vi "Source A.vi"() -> ()   [LabVIEW 2016, in "beamline sections.lvlib"]
doc: "This vi allows the user to control the beamline elements on the high voltage deck. It uses the GRoup3 controllers to access all three high voltage decks. The preacc and injector image faraday cup are controlled by the low end compact rio"
uses:
  controls/beamline sections.lvlib
  controls/SCA steerers.ctl
  save load/saveloadprev.ctl
  cRIO code/SCA/controls/SCA broadcast status.ctl
  save load/SaveLoad.lvlib
panel:
  in  "Tab Control":T1(tab)
  in  "Preview-Save-Load":T2
  out "Boolean":bool
  in  "Oven i":dbl
  in  "Y Steerer":dbl(slide) scale=-500.0..500.0
  in  "Pre-Acc":dbl(slide) scale=0.0..63.0
  in  "Einzel 2":dbl(slide) scale=0.0..10.0
  in  "X Steerer":dbl(slide) scale=-500.0..500.0
  in  "Einzel 1":dbl(slide) scale=0.0..12.0
  in  "Extractor":dbl(slide) scale=0.0..26.0
  in  "Immersion Lens":dbl(slide) scale=0.0..1.0
  out "Einzel 2 display":bool
  out "Cathode display":bool
  out "Oven display":bool
  out "Einzel 1 display":bool
  out "Immersion lens display":bool
  out "Steerer display":bool
  out "Pre acc display":bool=TRUE
  in  "Cathode V":dbl(slide) scale=0.0..12.0
  out "Cathode  cluster":T3 {"Cathode" format="%#_3g"; "Cathode\nVoltage" format="%#.2g"; "Cathode \nCurrent" format="%#.2g"}
  out "Extractor  cluster":T4 {"Extractor" format="%#_3g"; "Extractor \nVoltage" format="%#.2g"; "Extractor\n Current" format="%#.2g"}
  out "Immersion Lens  cluster":T5 {"Immersion Lens" format="%#_3g"; "Immersion Lens\nCurrent" format="%#.2g"; "Immersion Lens\nVoltage" format="%#.2g"}
  in  "stop":bool
  out "Oven cluster":T6 {"Oven V" format="%#.2g"; "Oven power" format="%#.2g"; "Oven  I readback" format="%#.2g"; "Oven Current\n Set point" format="%#.2g"}
  out "Einzel 1  cluster":T7 {"Einzel 1 Voltage" format="%#.2g"; "Einzel  Current" format="%#.2g"}
  out "Source Steerer cluster":T8 {"X steerer read" format="%#.2g"; "Y Steerer set" format="%#.2g"}
  out "Einzel 2  cluster":T9 {"Einzel 2 voltage" format="%#.2g"; "Einzel 2 Current" format="%#.2g"}
  out "Preacc cluster":T10 {"Pre-acc Voltage" format="%#.2g"; "Pre-acc current" format="%#.2g"}
  out "Cryo pump":T11
  out "Ion gauge Cluster 1":T12
  out "chop voltage":dbl
  in  "reset oven":bool
  out "Extractor display":bool
  in  "Cathode HV Enable":bool
  in  "Immersion HV Enable":bool
  in  "Extractor HV Enable":bool
  out "SCA Status":T13
  out "pre-acc set":dbl format="%#_3g"
  out "Pre-acc Voltage":dbl format="%#_3g"
  out "Pre-acc current":dbl format="%#_3g"
  out "inj cup out":bool
  out "Output Current":dbl format="%.4f"
  out "Output Power":dbl format="%.4f"
  out "Output Voltage":dbl format="%.4f"
  out "Read Set Current":dbl format="%.4f"
  out "Read Set Voltage":dbl format="%.4f"
  out "ID responce":string
  out "Address \"OK\"":string
  in  "Source A temp file":path=path "D:/Main Tune Parameters/Temp Configs/Source A.txt"
  out "Oven readback error":errorcluster
  out "SaveLoad error":errorcluster
  out "Oven Reset Error":errorcluster
  out "Oven Set Error":errorcluster
  out "SV error":errorcluster
  # "Source A"
  # "red is in the beamline\nblue is out of the beamline"
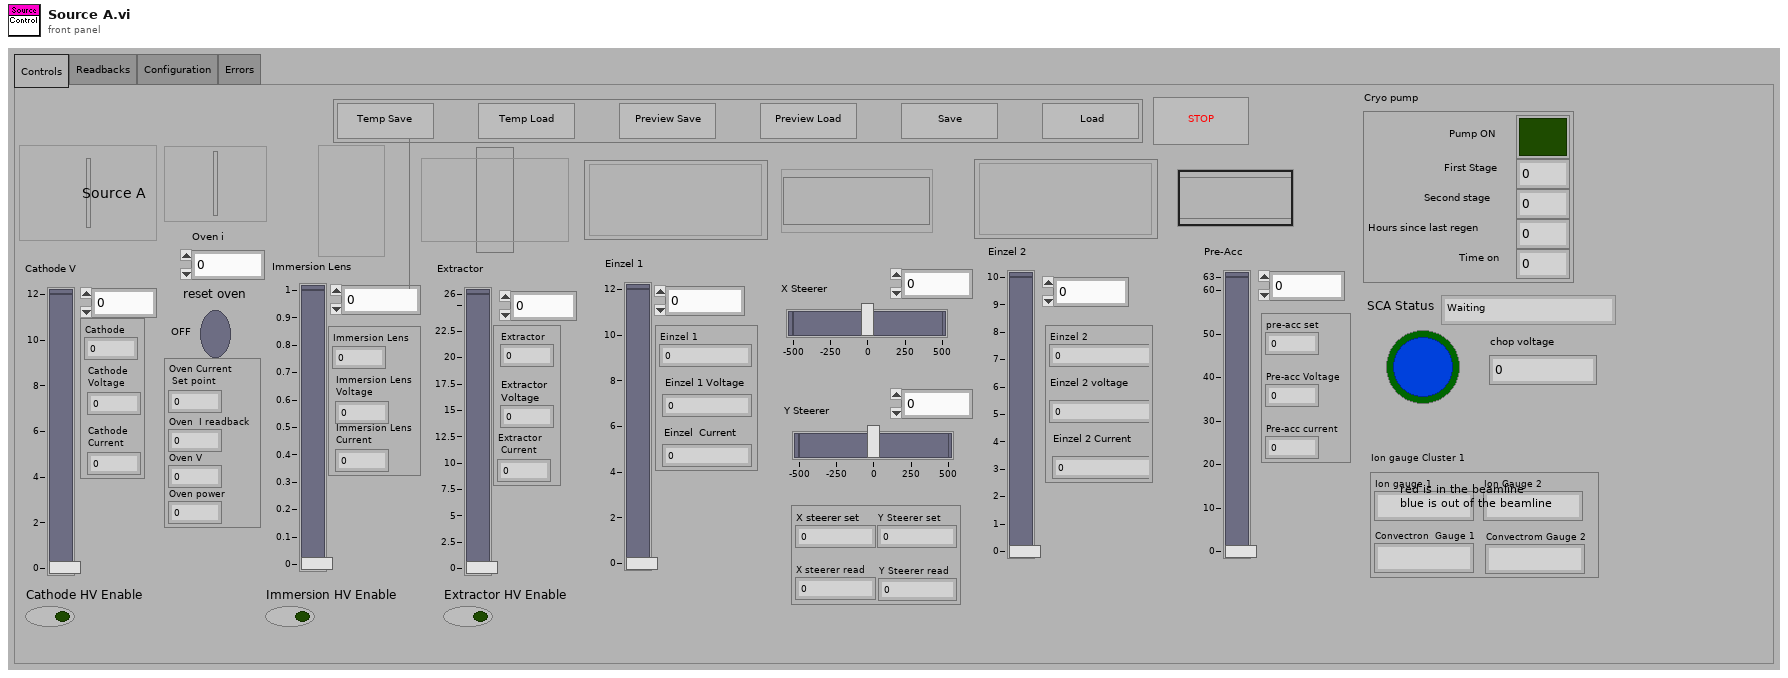
[diagram p1: front panel]
types:
  T1 = enum32{"Controls", "Readbacks", "Configuration", "Errors"}
  T2 = typedef "saveloadprev.ctl" = cluster{"Temp Save":bool, "Temp Load":bool, "Save":bool, "Load":bool, "Preview Save":bool, "Preview Load":bool}
  T3 = cluster{"Cathode":dbl, "Cathode\nVoltage":dbl, "Cathode \nCurrent":dbl}
  T4 = cluster{"Extractor":dbl, "Extractor \nVoltage":dbl, "Extractor\n Current":dbl}
  T5 = cluster{"Immersion Lens":dbl, "Immersion Lens\nCurrent":dbl, "Immersion Lens\nVoltage":dbl}
  T6 = cluster{"Oven  I readback":dbl, "Oven Current\n Set point":dbl, "Oven power":dbl, "Oven V ":dbl}
  T7 = cluster{"Einzel 1":dbl, "Einzel 1 Voltage":dbl, "Einzel  Current":dbl}
  T8 = typedef "SCA steerers.ctl" = cluster{"X steerer set":dbl, "X steerer read":dbl, "Y Steerer set":dbl, "Y Steerer read ":dbl}
  T9 = cluster{"Einzel 2":dbl, "Einzel 2 voltage":dbl, "Einzel 2 Current":dbl}
  T10 = cluster{"pre-acc set":dbl, "Pre-acc Voltage":dbl, "Pre-acc current":dbl}
  T11 = cluster{"First Stage":dbl, "Second stage":dbl, "Hours since last regen":dbl, "Pump ON":bool, "Time on":dbl}
  T12 = cluster{"Ion gauge 1":string, "Convectron  Gauge 1 ":string, "Ion Gauge 2":string, "Convectrom Gauge 2":string}
  T13 = typedef "SCA broadcast status.ctl" = enum16{"Waiting", "Changing samples", "Sample change complete", "Failure"}
  T14 = cluster{"Einzel 1":dbl, "Einzel 1\nVoltage":dbl, "Einzel \nCurrent":dbl}
  T15 = cluster{"Pre-Acc":dbl, "Double":dbl, "Double":dbl}
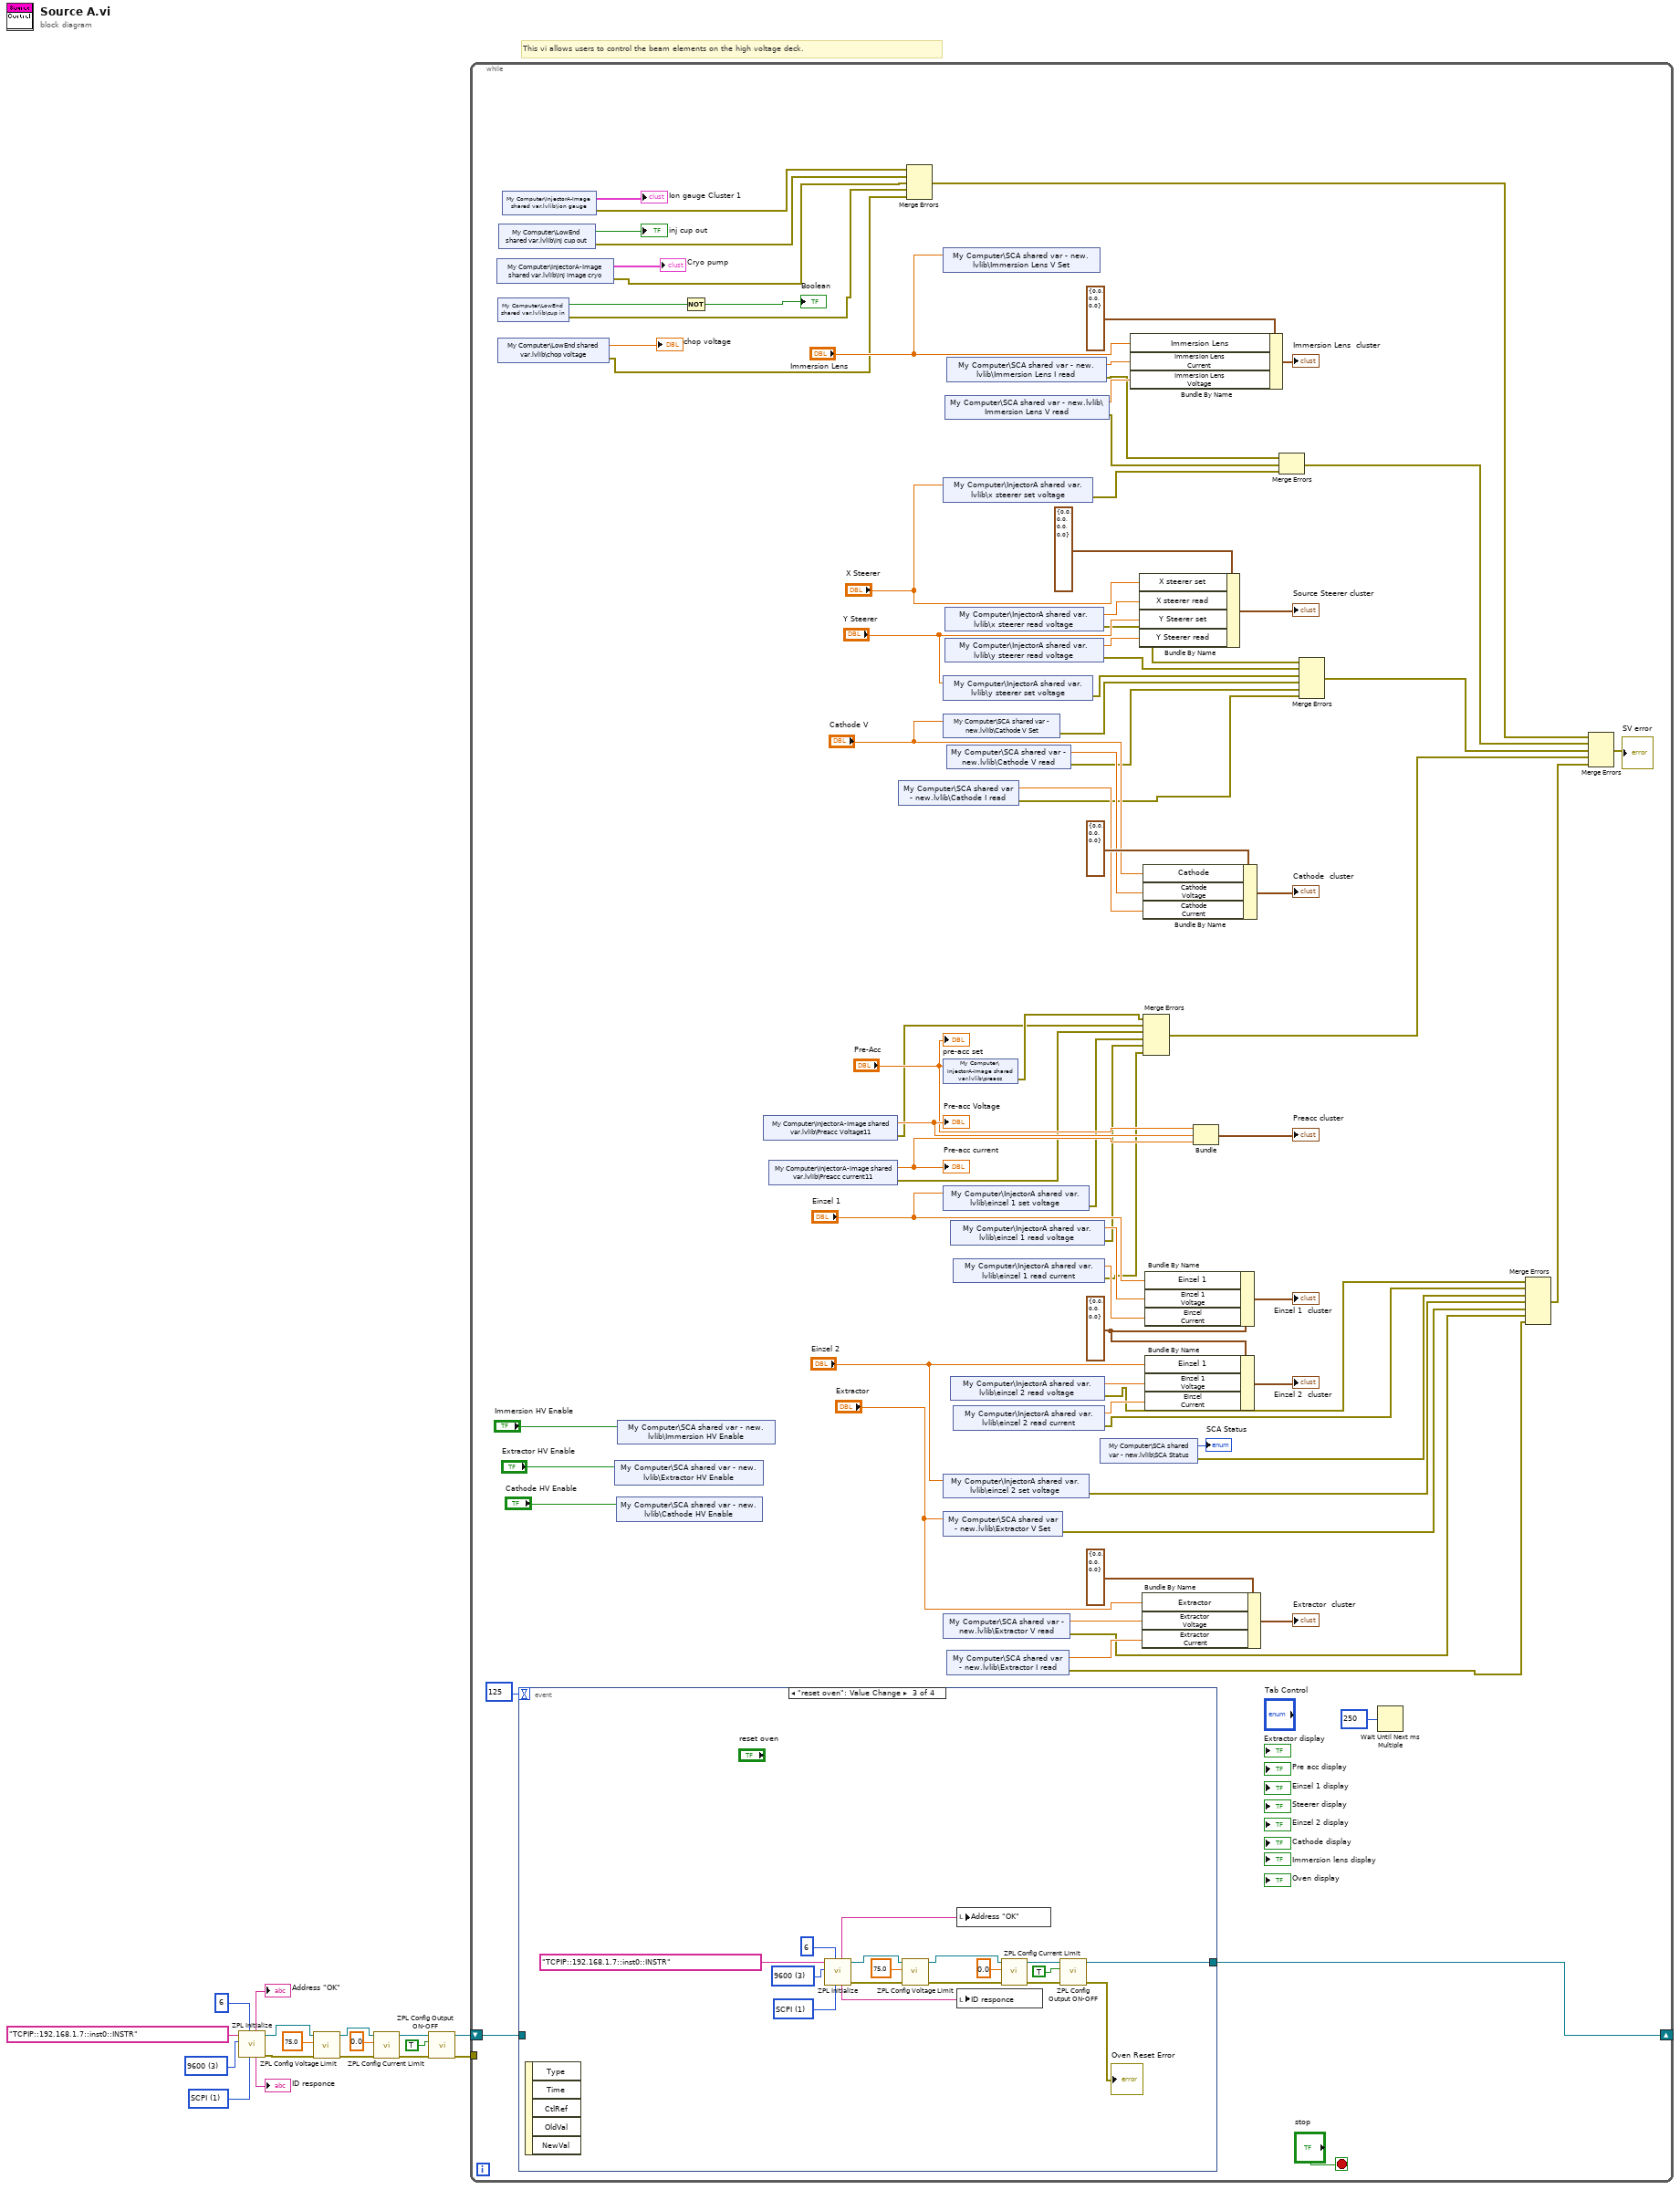
[diagram p0: block diagram]
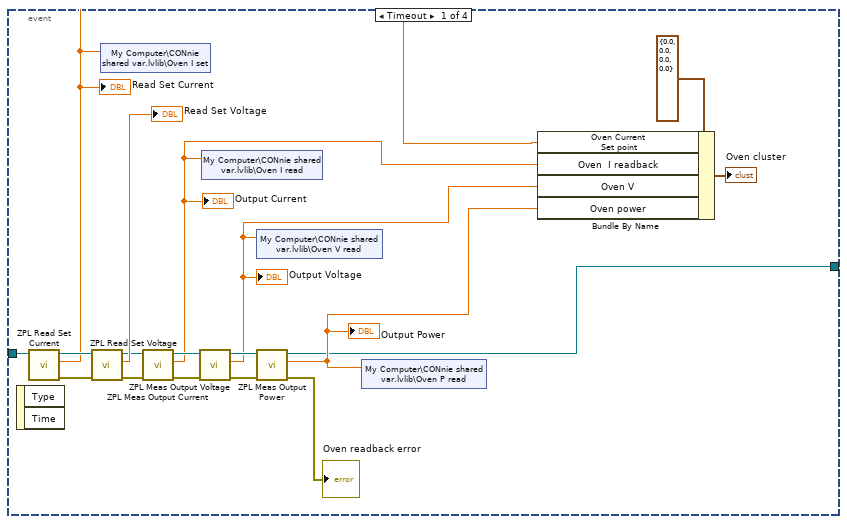
[diagram p2: hidden frame]
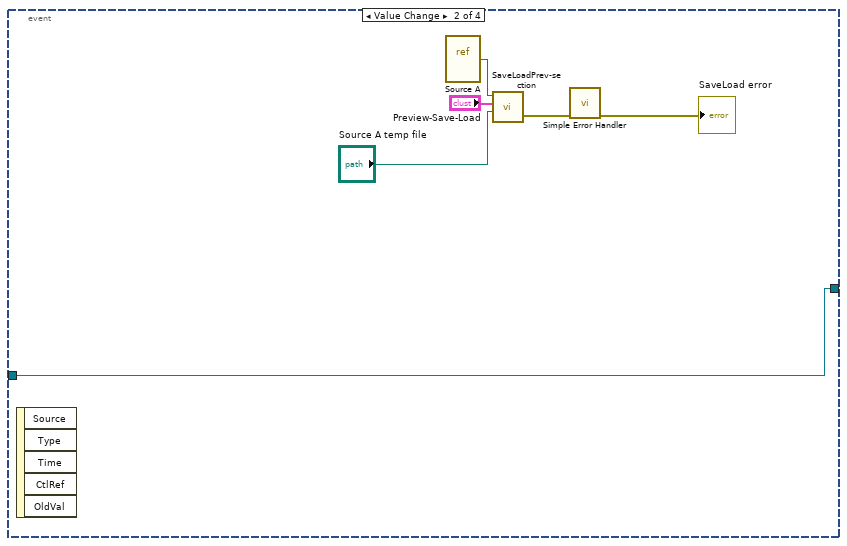
[diagram p3: hidden frame]
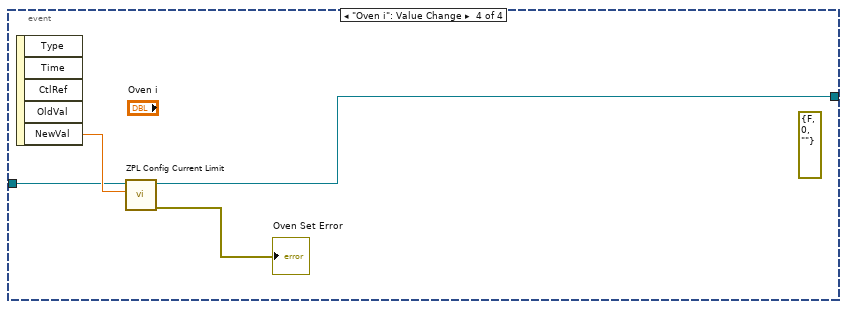
[diagram p4: hidden frame]
diagram:
  w17 = 3 items=["1200", "2400", "4800", "9600", "19200", "38400", "57600", "115200"] ("Baud Rate")
  w16 = i16 1 items=["GEN", "SCPI"] ("Language Selector")
  # "This vi allows users to control the beam elements on the high voltage deck."
  n1 = call "ZPL Initialize.vi"("Language Selector"=w16, "Address"=i16 6, "Baud Rate"=w17, "VISA"="TCPIP::192.168.1.7::inst0::INSTR" ("format string")) -> ("error out"=w7:errorcluster, "VISA  out"=w8:refnum<visa-resource-name>, "ID responce"=→"ID responce":string, "Address \"OK\""=→"Address \"OK\"":string)  [unwired: 4 in]
  n2 = call "ZPL Config Voltage Limit.vi"("error"=w7, "Voltage Limit"=75.0, "VISA"=w8) -> ("error out"=w9:errorcluster, "VISA out"=w10:refnum<visa-resource-name>)  [unwired: 7 in]
  n3 = call "ZPL Config Current Limit.vi"("error"=w9, "Current Limit"=0.0, "VISA"=w10) -> ("error out"=w13:errorcluster, "VISA out"=w12:refnum<visa-resource-name>)  [unwired: 7 in]
  n4 = call "ZPL Config Output ON-OFF.vi"("error"=w13, "Output ON"=TRUE, "VISA"=w12) -> ("error out"=w4:errorcluster, "VISA out"=w5:refnum<visa-resource-name>)  [unwired: 7 in]
  n5 = while {
    shift-right: [w22] -> _
    shift-left: w5 -> [w79]
    tunnel: w4 -> [_]
    stop <- "stop" stop-if-true
    w74 = T14 {"Einzel 1"=0.0, "Einzel 1\nVoltage"=0.0, "Einzel \nCurrent"=0.0} ("Einzel 1  cluster 2")
    n6 = shared-variable "My Computer\\InjectorA-Image shared var.lvlib\\inj image cryo"() -> (→"Cryo pump":T11, error out=w54:errorcluster)  [unwired: 1 in]
    n7 = shared-variable "My Computer\\LowEnd shared var.lvlib\\cup in"() -> (w93:bool, error out=w53:errorcluster)  [unwired: 1 in]
    n8 = shared-variable "My Computer\\LowEnd shared var.lvlib\\chop voltage"() -> (→"chop voltage":dbl, error out=w52:errorcluster)  [unwired: 1 in]
    n9 = shared-variable "My Computer\\LowEnd shared var.lvlib\\inj cup out"() -> (→"inj cup out":bool, error out=w55:errorcluster)  [unwired: 1 in]
    n10 = shared-variable "My Computer\\InjectorA-Image shared var.lvlib\\ion gauge"() -> (→"Ion gauge Cluster 1":cluster{string, string, string, string}, error out=w56:errorcluster)  [unwired: 1 in]
    n11 = event shown="[2] \"reset oven\": Value Change" {
      selector: _ -> [_ _ _ _]
      dyn-events: _ -> [_ _ _ _]
      timeout: 125 -> [_ _ _ _]
      tunnel: w79 -> [w108 w118 _ w143]
      tunnel: [w101 w118 w124 w141] -> w22
      event Timeout {
        n12 = event-data() -> ()  [unwired: 1 in, 2 out]
        n13 = call "ZPL Read Set Current.vi"("VISA"=w108) -> ("error out"=w117:errorcluster, "Read Set Current"=w104:dbl, "VISA out"=w116:refnum<visa-resource-name>)  [unwired: 8 in]
        "Read Set Current" <- w104
        n14 = call "ZPL Read Set Voltage.vi"("error"=w117, "VISA"=w116) -> ("error out"=w113:errorcluster, "Read Set Voltage"=→"Read Set Voltage":dbl, "VISA out"=w114:refnum<visa-resource-name>)  [unwired: 7 in]
        n15 = shared-variable "My Computer\\CONnie shared var.lvlib\\Oven I set"(w104) -> ()  [unwired: 1 in, 1 out]
        n16 = call "ZPL Meas Output Current.vi"("error"=w113, "VISA"=w114) -> ("error out"=w111:errorcluster, "Output Current"=w105:dbl, "VISA out"=w112:refnum<visa-resource-name>)  [unwired: 7 in]
        "Output Current" <- w105
        n17 = call "ZPL Meas Output Voltage.vi"("error"=w111, "VISA"=w112) -> ("error out"=w109:errorcluster, "Output Voltage"=w103:dbl, "VISA out"=w110:refnum<visa-resource-name>)  [unwired: 7 in]
        "Output Voltage" <- w103
        n18 = shared-variable "My Computer\\CONnie shared var.lvlib\\Oven I read"(w105) -> ()  [unwired: 1 in, 1 out]
        n19 = shared-variable "My Computer\\CONnie shared var.lvlib\\Oven V read"(w103) -> ()  [unwired: 1 in, 1 out]
        n20 = call "ZPL Meas Output Power.vi"("error"=w109, "VISA"=w110) -> ("error out"=→"Oven readback error":errorcluster, "Output Power"=w102:dbl, "VISA out"=w101:refnum<visa-resource-name>)  [unwired: 7 in]
        "Output Power" <- w102
        n21 = shared-variable "My Computer\\CONnie shared var.lvlib\\Oven P read"(w102) -> ()  [unwired: 1 in, 1 out]
        n22 = Bundle By Name(cluster=T6 {"Oven  I readback"=0.0, "Oven Current\n Set point"=0.0, "Oven power"=0.0, "Oven V "=0.0} ("Oven cluster"), "Oven Current\n Set point"=w104, "Oven  I readback"=w105, "Oven V"=w103, "Oven power"=w102) -> (→"Oven cluster":T6)
      }
      event Value Change {
        n23 = event-data() -> ()  [unwired: 1 in, 5 out]
        n24 = vi-ref "Source A.vi"() -> (w121:refnum<vi>)
        n25 = call "SaveLoadPrev-section.vi"("file path (use dialog)"="Source A temp file", "Cluster 2"="Preview-Save-Load", "VI Refnum"=w121) -> ("error out"=w120:errorcluster)  [unwired: 2 in]
        n26 = call <vilib>:"Simple Error Handler.vi"("error in (no error)"=w120) -> ("error out"=→"SaveLoad error":errorcluster)  [unwired: 4 in, 4 out]
      }
      event "reset oven": Value Change {
        w129 = 3 items=["1200", "2400", "4800", "9600", "19200", "38400", "57600", "115200"] ("Baud Rate")
        w130 = i16 1 items=["GEN", "SCPI"] ("Language Selector")
        n27 = event-data() -> ()  [unwired: 1 in, 5 out]
        n28 = call "ZPL Initialize.vi"("Language Selector"=w130, "Address"=i16 6, "Baud Rate"=w129, "VISA"="TCPIP::192.168.1.7::inst0::INSTR" ("format string")) -> ("error out"=w138:errorcluster, "VISA  out"=w137:refnum<visa-resource-name>, "ID responce"=w126:string, "Address \"OK\""=w127:string)  [unwired: 4 in]
        n29 = call "ZPL Config Voltage Limit.vi"("error"=w138, "Voltage Limit"=75.0, "VISA"=w137) -> ("error out"=w136:errorcluster, "VISA out"=w135:refnum<visa-resource-name>)  [unwired: 7 in]
        n30 = local write "Address \"OK\""(w127) -> ()
        n31 = local write "ID responce"(w126) -> ()
        n32 = call "ZPL Config Current Limit.vi"("error"=w136, "Current Limit"=0.0, "VISA"=w135) -> ("error out"=w132:errorcluster, "VISA out"=w133:refnum<visa-resource-name>)  [unwired: 7 in]
        n33 = call "ZPL Config Output ON-OFF.vi"("error"=w132, "Output ON"=TRUE, "VISA"=w133) -> ("error out"=→"Oven Reset Error":errorcluster, "VISA out"=w124:refnum<visa-resource-name>)  [unwired: 7 in]
      }
      event "Oven i": Value Change {
        (unwired) errorcluster {"status"=FALSE, "code"=0, "source"=""} ("error constant")
        n34 = event-data() -> ("NewVal"=w144:dbl)  [unwired: 1 in, 4 out]
        n35 = call "ZPL Config Current Limit.vi"("Current Limit"=w144, "VISA"=w143) -> ("error out"=→"Oven Set Error":errorcluster, "VISA out"=w141:refnum<visa-resource-name>)  [unwired: 8 in]
      }
    }
    n36 = shared-variable "My Computer\\SCA shared var - new.lvlib\\Extractor HV Enable"("Extractor HV Enable") -> ()  [unwired: 1 in, 1 out]
    n37 = shared-variable "My Computer\\SCA shared var - new.lvlib\\Cathode HV Enable"("Cathode HV Enable") -> ()  [unwired: 1 in, 1 out]
    n38 = shared-variable "My Computer\\SCA shared var - new.lvlib\\Immersion HV Enable"("Immersion HV Enable") -> ()  [unwired: 1 in, 1 out]
    n39 = Not(x=w93) -> (.not. x?=→"Boolean":bool)
    n40 = shared-variable "My Computer\\InjectorA-Image shared var.lvlib\\Preacc Voltage11"() -> (w60:dbl, error out=w38:errorcluster)  [unwired: 1 in]
    "Pre-acc Voltage" <- w60
    n41 = shared-variable "My Computer\\InjectorA-Image shared var.lvlib\\Preacc current11"() -> (w58:dbl, error out=w37:errorcluster)  [unwired: 1 in]
    "Pre-acc current" <- w58
    n42 = shared-variable "My Computer\\SCA shared var - new.lvlib\\Cathode I read"() -> (w81:dbl, error out=w43:errorcluster)  [unwired: 1 in]
    n43 = Merge Errors(w56, w55, w54, w53, w52) -> (w42:errorcluster)
    n44 = shared-variable "My Computer\\SCA shared var - new.lvlib\\Immersion Lens V Set"("Immersion Lens") -> ()  [unwired: 1 in, 1 out]
    n45 = shared-variable "My Computer\\InjectorA shared var.lvlib\\x steerer set voltage"("X Steerer") -> (error out=w49:errorcluster)  [unwired: 1 in]
    n46 = shared-variable "My Computer\\InjectorA shared var.lvlib\\y steerer set voltage"("Y Steerer") -> (error out=w46:errorcluster)  [unwired: 1 in]
    n47 = shared-variable "My Computer\\SCA shared var - new.lvlib\\Cathode V Set"("Cathode V") -> (error out=w45:errorcluster)  [unwired: 1 in]
    n48 = shared-variable "My Computer\\InjectorA-Image shared var.lvlib\\preacc"("Pre-Acc") -> (error out=w39:errorcluster)  [unwired: 1 in]
    n49 = shared-variable "My Computer\\InjectorA shared var.lvlib\\einzel 1 set voltage"("Einzel 1") -> (error out=w36:errorcluster)  [unwired: 1 in]
    n50 = shared-variable "My Computer\\InjectorA shared var.lvlib\\einzel 2 set voltage"("Einzel 2") -> (error out=w29:errorcluster)  [unwired: 1 in]
    n51 = shared-variable "My Computer\\SCA shared var - new.lvlib\\Extractor V Set"("Extractor") -> (error out=w28:errorcluster)  [unwired: 1 in]
    n52 = shared-variable "My Computer\\SCA shared var - new.lvlib\\Extractor V read"() -> (w87:dbl, error out=w27:errorcluster)  [unwired: 1 in]
    n53 = shared-variable "My Computer\\SCA shared var - new.lvlib\\Immersion Lens V read"() -> (w61:dbl, error out=w50:errorcluster)  [unwired: 1 in]
    n54 = shared-variable "My Computer\\InjectorA shared var.lvlib\\x steerer read voltage"() -> (w67:dbl, error out=w48:errorcluster)  [unwired: 1 in]
    n55 = shared-variable "My Computer\\InjectorA shared var.lvlib\\y steerer read voltage"() -> (w65:dbl, error out=w47:errorcluster)  [unwired: 1 in]
    n56 = shared-variable "My Computer\\SCA shared var - new.lvlib\\Immersion Lens I read"() -> (w62:dbl, error out=w51:errorcluster)  [unwired: 1 in]
    n57 = shared-variable "My Computer\\SCA shared var - new.lvlib\\Cathode V read"() -> (w82:dbl, error out=w44:errorcluster)  [unwired: 1 in]
    n58 = shared-variable "My Computer\\SCA shared var - new.lvlib\\Extractor I read"() -> (w85:dbl, error out=w26:errorcluster)  [unwired: 1 in]
    n59 = shared-variable "My Computer\\InjectorA shared var.lvlib\\einzel 1 read voltage"() -> (w78:dbl, error out=w35:errorcluster)  [unwired: 1 in]
    n60 = shared-variable "My Computer\\InjectorA shared var.lvlib\\einzel 2 read voltage"() -> (w71:dbl, error out=w32:errorcluster)  [unwired: 1 in]
    n61 = shared-variable "My Computer\\InjectorA shared var.lvlib\\einzel 1 read current"() -> (w77:dbl, error out=w34:errorcluster)  [unwired: 1 in]
    n62 = shared-variable "My Computer\\InjectorA shared var.lvlib\\einzel 2 read current"() -> (w70:dbl, error out=w31:errorcluster)  [unwired: 1 in]
    n63 = shared-variable "My Computer\\SCA shared var - new.lvlib\\SCA Status"() -> (→"SCA Status":T13, error out=w30:errorcluster)  [unwired: 1 in]
    n64 = Bundle By Name(cluster=T5 {"Immersion Lens"=0.0, "Immersion Lens\nCurrent"=0.0, "Immersion Lens\nVoltage"=0.0} ("Immersion Lens  cluster  2"), "Immersion Lens"="Immersion Lens", "Immersion Lens\nCurrent"=w62, "Immersion Lens\nVoltage"=w61) -> (→"Immersion Lens  cluster":T5)
    n65 = Bundle By Name(cluster=T8 {"X steerer set"=0.0, "X steerer read"=0.0, "Y Steerer set"=0.0, "Y Steerer read "=0.0} ("Source Steerer cluster 2"), "X steerer set"="X Steerer", "X steerer read"=w67, "Y Steerer set"="Y Steerer", "Y Steerer read"=w65) -> (→"Source Steerer cluster":T8)
    n66 = Bundle By Name(cluster=T4 {"Extractor"=0.0, "Extractor \nVoltage"=0.0, "Extractor\n Current"=0.0} ("Extractor  cluster"), "Extractor"="Extractor", "Extractor \nVoltage"=w87, "Extractor\n Current"=w85) -> (→"Extractor  cluster":T4)
    n67 = Bundle By Name(cluster=T3 {"Cathode"=0.0, "Cathode\nVoltage"=0.0, "Cathode \nCurrent"=0.0} ("Cathode  cluster"), "Cathode"="Cathode V", "Cathode\nVoltage"=w82, "Cathode \nCurrent"=w81) -> (→"Cathode  cluster":T3)
    n68 = Merge Errors(w39, w38, w37, w36, w35, w34) -> (w33:errorcluster)
    n69 = Bundle By Name(cluster=w74, "Einzel 1"="Einzel 1", "Einzel 1\nVoltage"=w78, "Einzel \nCurrent"=w77) -> (→"Einzel 1  cluster":T14)
    n70 = Bundle By Name(cluster=w74, "Einzel 1"="Einzel 2", "Einzel 1\nVoltage"=w71, "Einzel \nCurrent"=w70) -> (→"Einzel 2  cluster":T14)
    n71 = Bundle("Pre-Acc"="Pre-Acc", "Double"=w60, "Double"=w58) -> (→"Preacc cluster":T15)  [unwired: 1 out]
    n72 = Merge Errors(w51, w50, w49) -> (w41:errorcluster)
    n73 = Merge Errors(w48, w47, w46, w45, w44, w43) -> (w40:errorcluster)
    n74 = Wait Until Next ms Multiple(millisecond multiple=u32 250) -> ()  [unwired: 1 out]
    n75 = Merge Errors(w32, w31, w30, w29, w28, w27, w26) -> (w25:errorcluster)
    n76 = Merge Errors(w42, w41, w40, w33, w25) -> (→"SV error":errorcluster)
    "pre-acc set" <- "Pre-Acc"
  }
